vi "display_image.vi"(8 "error in":errorcluster, 11 "file_name":string="shell_volume.png") -> (0 "error out":errorcluster, 3 "status":bool, 4 "path":path)   [LabVIEW 2019]
panel:
  in  "command":string="rundll32 \"C:\\Program Files\\Windows Photo Viewer\\PhotoViewer.dll\",ImageView_Fullscreen"
  # "Sub-VI to play a WAV file."
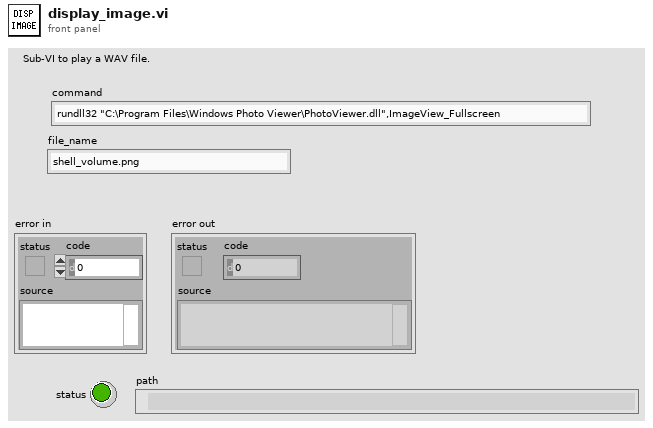
[diagram p1: front panel]
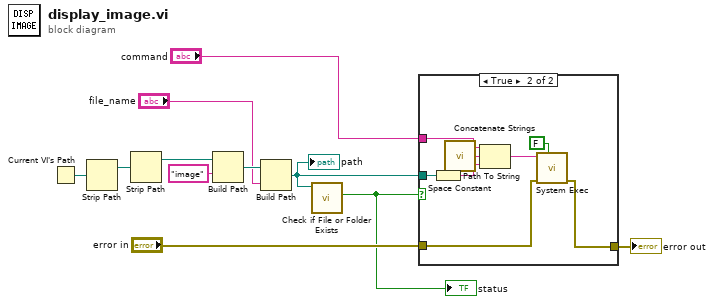
[diagram p0: block diagram]
diagram:
  n1 = Current VI's Path() -> (path=w7:path)
  n2 = Strip Path(path=w7) -> (stripped path=w2:path)  [unwired: 1 out]
  n3 = Strip Path(path=w2) -> (stripped path=w1:path)  [unwired: 1 out]
  n4 = Build Path(base path=w1, name or relative path="image") -> (appended path=w5:path)
  n5 = Build Path(base path=w5, name or relative path="file_name") -> (appended path=w8:path)
  "path" <- w8
  n6 = call <vilib>:"Check if File or Folder Exists.vi"("path"=w8) -> ("file or folder exists?"=w9:bool)  [unwired: 8 in, 2 out]
  "status" <- w9
  n7 = case shown="True" w9 {
    tunnel: "error in" -> [w12 w15]
    tunnel: [w12 w14] -> w10
    tunnel: w8 -> [_ w20]
    tunnel: "command" -> [_ w17]
    frame False {
    }
    frame True {
      n8 = Path To String(path=w20) -> (string=w19:string)
      n9 = call <vilib>:"Space Constant.vi"() -> ("String"=w18:string)
      n10 = Concatenate Strings(w17, w18, w19) -> (w16:string)
      n11 = call <vilib>:"System Exec.vi"("wait until completion? (T)"=FALSE, "error in (no error)"=w15, "command line"=w16) -> ("error out"=w14:errorcluster)  [unwired: 5 in, 3 out]
    }
  }
  "error out" <- w10
